vi "Differential IO.vi"(8 "error in (no error)":errorcluster, 11 "Node Ptr":T4 format="%.0x") -> (0 "error out":errorcluster)   [LabVIEW 2016, in "DCM System Explorer.lvlib"]
uses:
  DCM System Explorer.lvlib
  <vilib>/NI Veristand/Custom Device API/Custom Device Item Ref.ctl
  <vilib>/Powertrain Controls/Device Drivers/DCM/Diff IO/RT/Setup.ctl
  <vilib>/Powertrain Controls/Device Drivers/DCM/Diff IO/FPGA/Mode.ctl
  <vilib>/Powertrain Controls/Device Drivers/DCM/Diff IO/RT/Angle Control.ctl
  Shared/DCM Properties.vi
  <vilib>/NI Veristand/Custom Device API/Get Item Property (String Array).vi
  <vilib>/NI Veristand/Custom Device API/Get Item Property (Double Array).vi
  Shared/DCM Constants and GUIDs.vi
  <vilib>/NI Veristand/Custom Device API/Set Item Property (String Array).vi
  <vilib>/NI Veristand/Custom Device API/Set Item Property (Double Array).vi
  <vilib>/NI VeriStand/Custom Device API/Custom Device API.lvlib
  DCM Shared.lvlib
  <vilib>/Powertrain Controls/Device Drivers/DCM/Diff IO/FPGA/DCM - FPGA - Diff IO.lvlib
  <vilib>/Powertrain Controls/Device Drivers/DCM/Diff IO/RT/DCM - RT - Diff IO.lvlib
panel:
  in  "Digital filter [s]":sgl format="%#_2p"
  in  "Filters":sgl[](array[numeric])
  in  "_Setup Element":T1={"Mode"=enum."Off", "Capture Start [DBTDC]"=0.0, "Capture End [DBTDC]"=0.0, "Invert"=FALSE, "Frequency [Hz]"=0.0, "Duty Cycle [%]"=0.0, "TDC Offset [CAD]"=0.0, "Window Start [DBTDC]"=0.0, "Window End [DBTDC]"=0.0, "Angles"=[{"Enable"=FALSE, "Location [DBTDC]"=0.0, "Duration [s]"=0.0}, {"Enable"=FALSE, "Location [DBTDC]"=0.0, "Duration [s]"=0.0}, {"Enable"=FALSE, "Location [DBTDC]"=0.0, "Duration [s]"=0.0}, {"Enable"=FALSE, "Location [DBTDC]"=0.0, "Duration [s]"=0.0}], "Skip Fire"=FALSE, "Skip Fire Index"=0} caption="Command Setup" {"Skip Fire Index" max=7; "Angles"."Duration [s]" format="%#_3p"; "Frequency [Hz]" format="%#_3p"}
  in  "_Refresh":bool
  in  "Channel Names":string[](array[string])=["", "", "", "", "", "", "", "", "", "", "", ""]
  in  "Channel Name":string
  in  "_DiffIO Channels":i32[](listbox) caption="Channel Summary"
  in  "_Save Changes?":bool
  in  "Setup":T1[](array[typedef]) caption="Differential I/O Setup" {"Skip Fire Index" max=7; "Angles"."Duration [s]" format="%#_3p"; "Frequency [Hz]" format="%#_3p"}
  in  "Header":cluster{"Section Name":string}={"Section Name"="Differential I/O Initial Settings"}
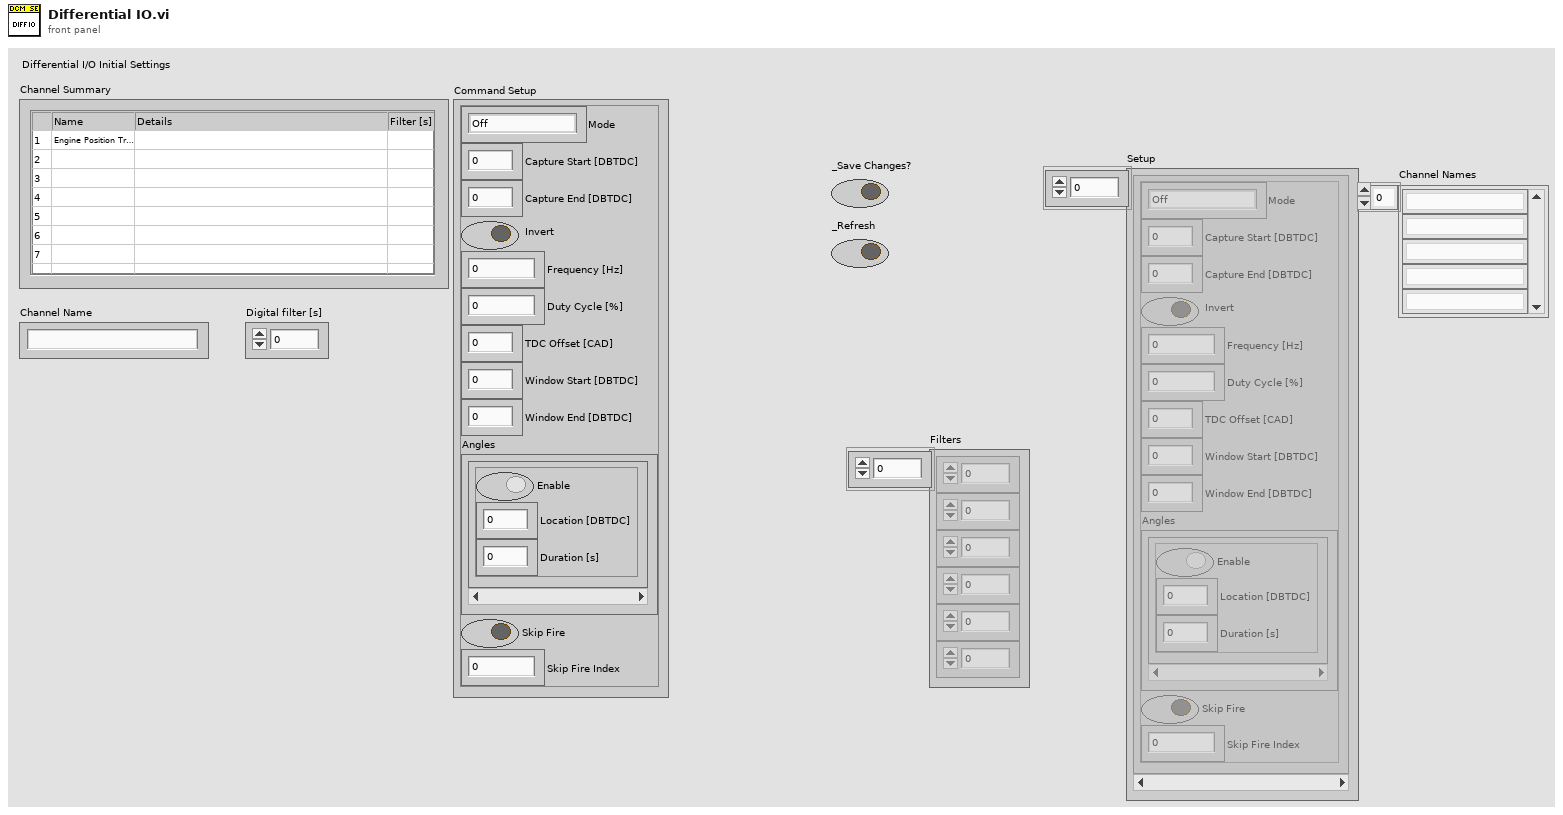
[diagram p1: front panel]
types:
  T1 = typedef "DCM - RT - Diff IO.lvlib/Setup.ctl" = cluster{"Mode":T2, "Capture Start [DBTDC]":sgl, "Capture End [DBTDC]":sgl, "Invert":bool, "Frequency [Hz]":sgl, "Duty Cycle [%]":sgl, "TDC Offset [CAD]":sgl, "Window Start [DBTDC]":sgl, "Window End [DBTDC]":sgl, "Angles":T3[], "Skip Fire":bool, "Skip Fire Index":u8}
  T2 = typedef "DCM - FPGA - Diff IO.lvlib/Mode.ctl" = enum8{"Off", "Input", "Pulse Width Modulation", "Engine Position Tracking", "Serial Out 1", "Serial Out 2", "EPTx Sync"}
  T3 = typedef "DCM - RT - Diff IO.lvlib/Angle Control.ctl" = cluster{"Enable":bool, "Location [DBTDC]":sgl, "Duration [s]":sgl}
  T4 = typedef "Custom Device API.lvlib/Custom Device Item Ref.ctl" = u64
  T5 = typedef "Custom Device API.lvlib/Custom Device Commands.ctl" = enum16{"Default", "Item renamed", "Shutdown", "Dynamic button pressed"}
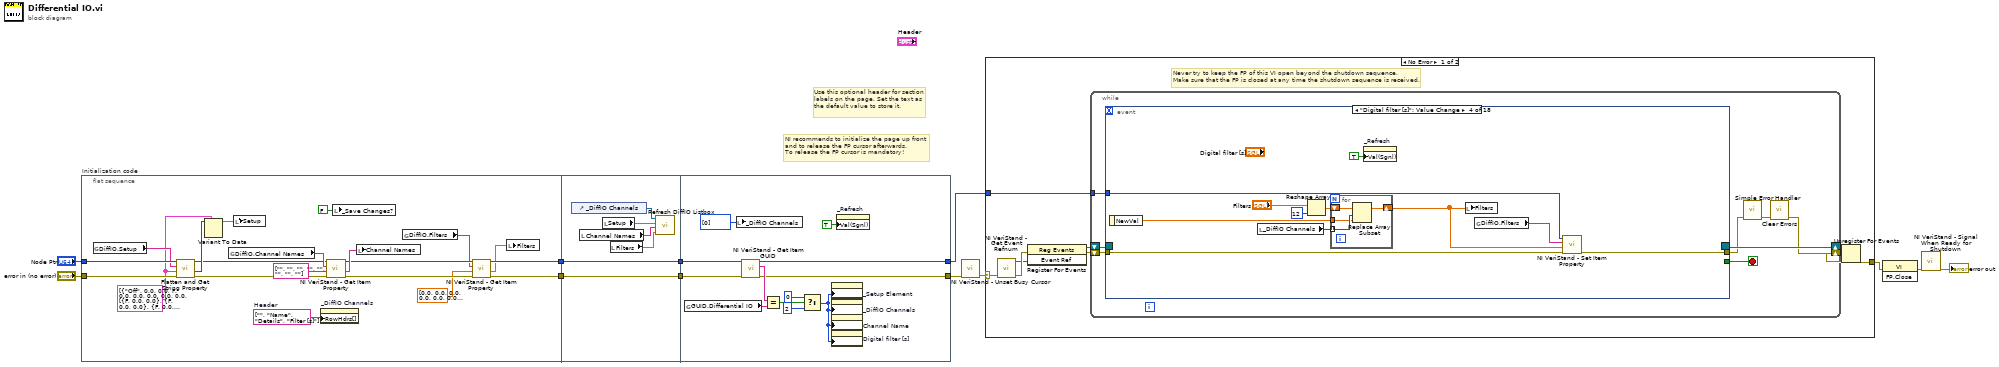
[diagram p0: block diagram]
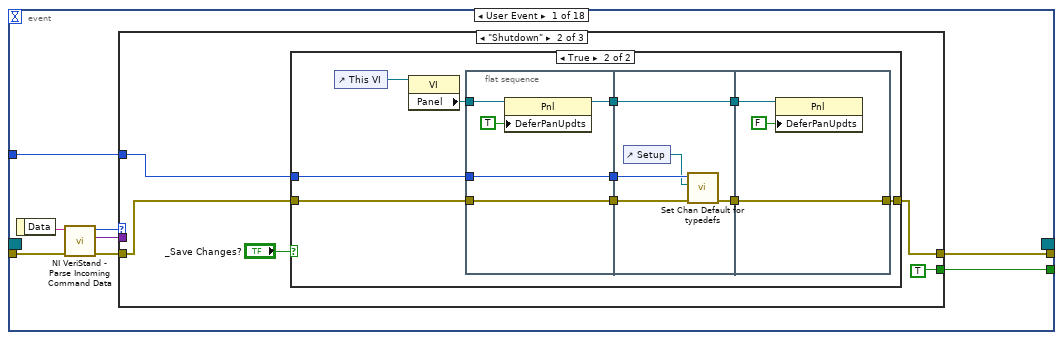
[diagram p2: hidden frame]
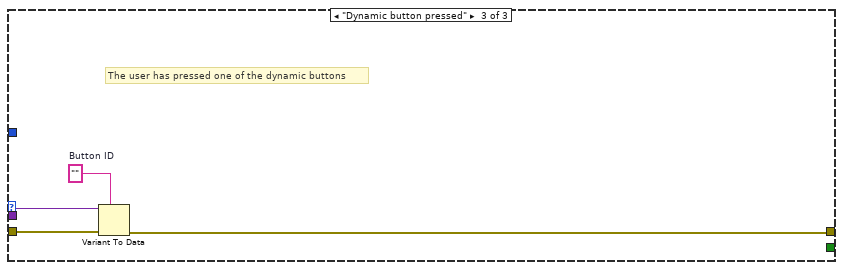
[diagram p5: hidden frame]
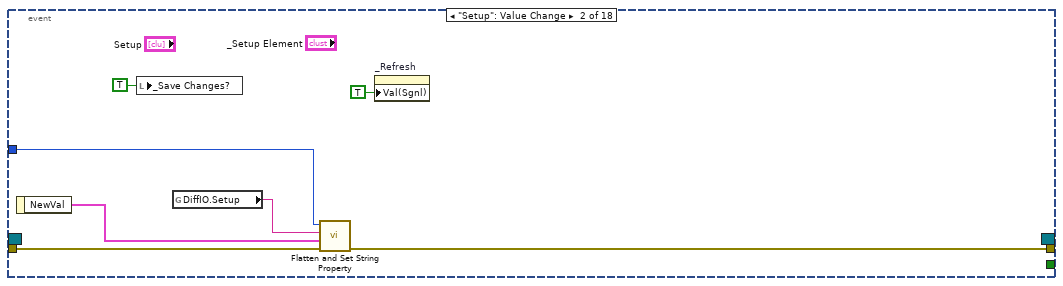
[diagram p6: hidden frame]
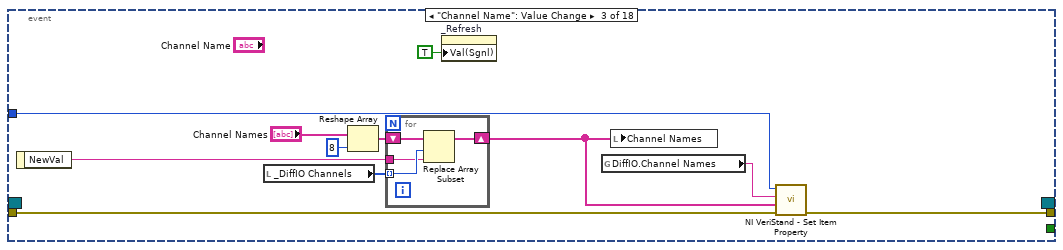
[diagram p7: hidden frame]
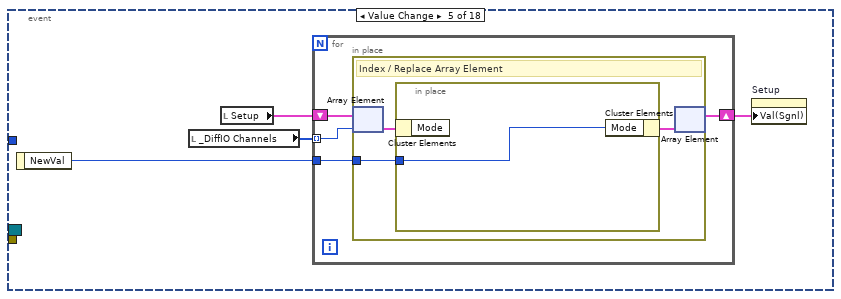
[diagram p8: hidden frame]
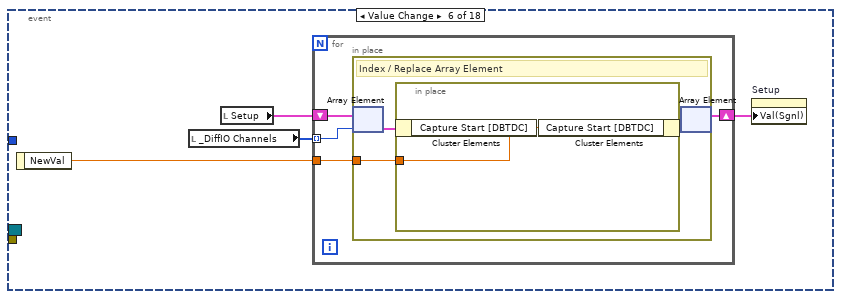
[diagram p9: hidden frame]
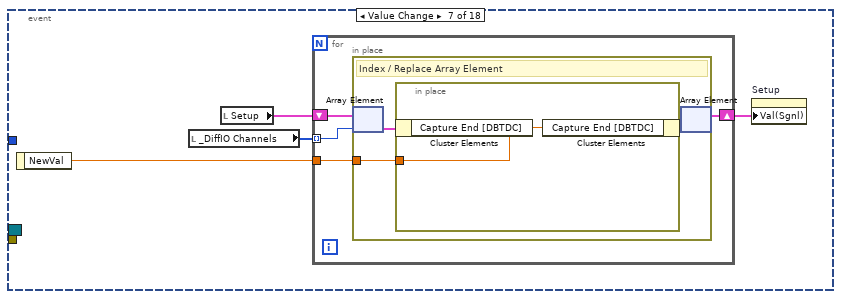
[diagram p10: hidden frame]
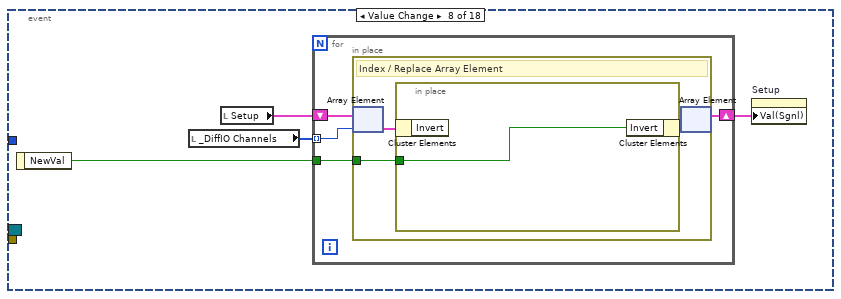
[diagram p11: hidden frame]
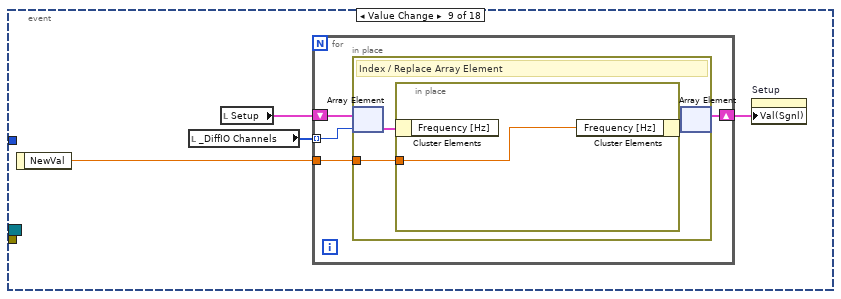
[diagram p12: hidden frame]
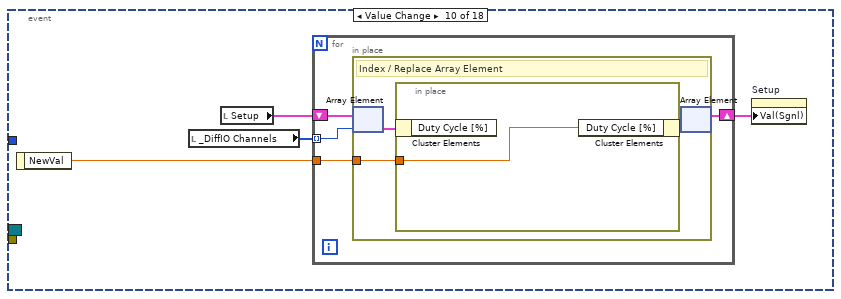
[diagram p13: hidden frame]
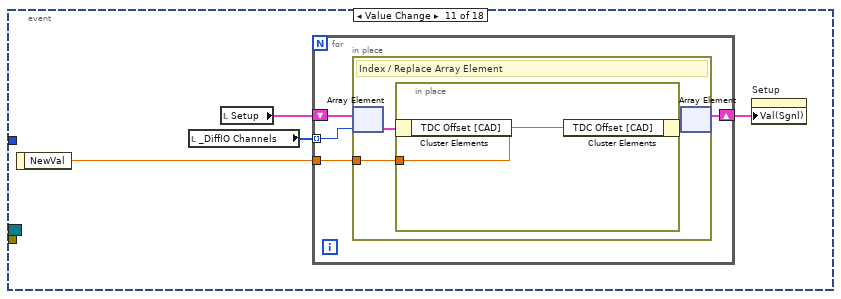
[diagram p14: hidden frame]
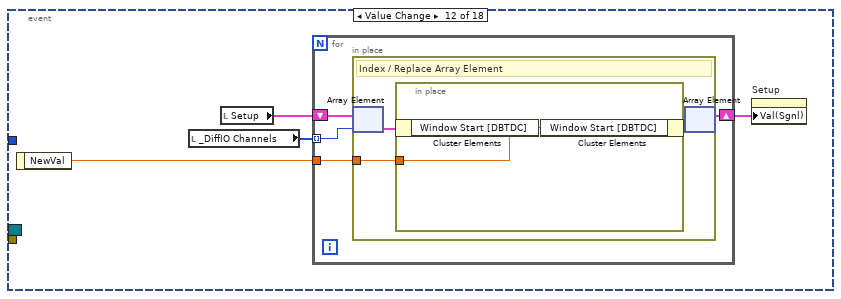
[diagram p15: hidden frame]
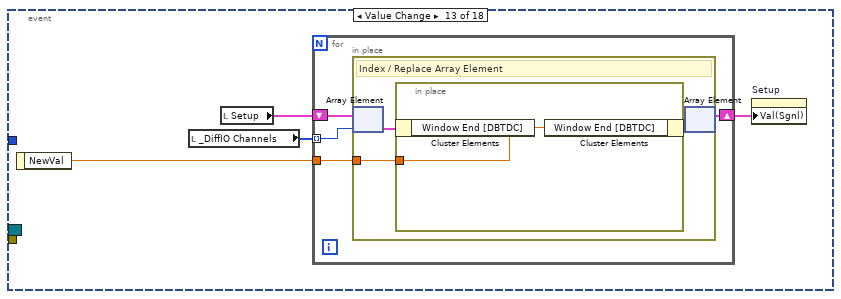
[diagram p16: hidden frame]
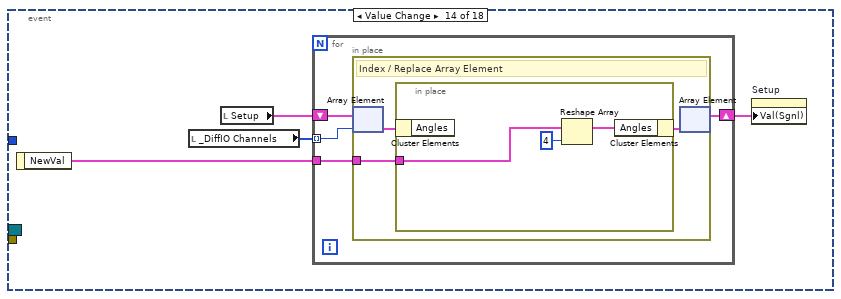
[diagram p17: hidden frame]
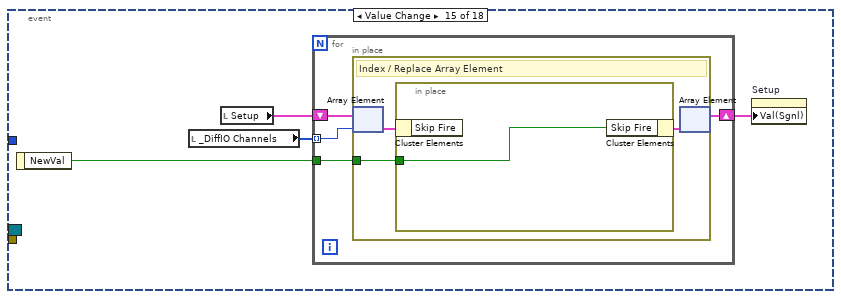
[diagram p18: hidden frame]
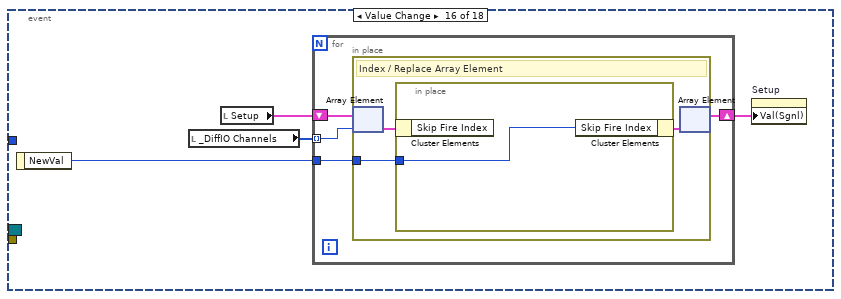
[diagram p19: hidden frame]
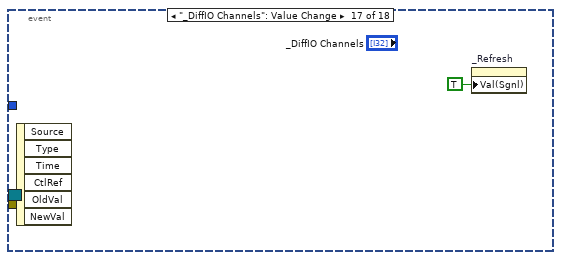
[diagram p20: hidden frame]
diagram:
  # "Use this optional header for section labels on the page. Set the text as the default value to store it."
  # "NI recommends to initialize the page up front\nand to release the FP cursor afterwards.\nTo release the FP cursor is mandatory!"
  n1 = flat-sequence "Initialization code" {
    tunnel: "Node Ptr" -> [w30]
    tunnel: "error in (no error)" -> [w31]
    tunnel: [w17] -> w5
    tunnel: [w16] -> w1
    tunnel: w5 -> [w37]
    tunnel: [w38] -> w4
    tunnel: [w37] -> w3
    tunnel: w1 -> [w38]
    tunnel: [w43] -> w2
    tunnel: [w42] -> w6
    tunnel: w4 -> [w45]
    tunnel: w3 -> [w44]
    frame #0 {
      w22 = string[] ["", "Name", "Details", "Filter [s]"]  # Header
      w28 = T1[] [{"Mode"=enum."Off", "Capture Start [DBTDC]"=0.0, "Capture End [DBTDC]"=0.0, "Invert"=FALSE, "Frequency [Hz]"=0.0, "Duty Cycle [%]"=0.0, "TDC Offset [CAD]"=0.0, "Window Start [DBTDC]"=0.0, "Window End [DBTDC]"=0.0, "Angles"=[{"Enable"=FALSE, "Location [DBTDC]"=0.0, "Duration [s]"=0.0}, {"Enable"=FALSE, "Location [DBTDC]"=0.0, "Duration [s]"=0.0}, {"Enable"=FALSE, "Location [DBTDC]"=0.0, "Duration [s]"=0.0}, {"Enable"=FALSE, "Location [DBTDC]"=0.0, "Duration [s]"=0.0}], "Skip Fire"=FALSE, "Skip Fire Index"=0}, {"Mode"=enum."Off", "Capture Start [DBTDC]"=0.0, "Capture End [DBTDC]"=0.0, "Invert"=FALSE, "Frequency [Hz]"=0.0, "Duty Cycle [%]"=0.0, "TDC Offset [CAD]"=0.0, "Window Start [DBTDC]"=0.0, "Window End [DBTDC]"=0.0, "Angles"=[{"Enable"=FALSE, "Location [DBTDC]"=0.0, "Duration [s]"=0.0}, {"Enable"=FALSE, "Location [DBTDC]"=0.0, "Duration [s]"=0.0}, {"Enable"=FALSE, "Location [DBTDC]"=0.0, "Duration [s]"=0.0}, {"Enable"=FALSE, "Location [DBTDC]"=0.0, "Duration [s]"=0.0}], "Skip Fire"=FALSE, "Skip Fire Index"=0}, {"Mode"=enum."Off", "Capture Start [DBTDC]"=0.0, "Capture End [DBTDC]"=0.0, "Invert"=FALSE, "Frequency [Hz]"=0.0, "Duty Cycle [%]"=0.0, "TDC Offset [CAD]"=0.0, "Window Start [DBTDC]"=0.0, "Window End [DBTDC]"=0.0, "Angles"=[{"Enable"=FALSE, "Location [DBTDC]"=0.0, "Duration [s]"=0.0}, {"Enable"=FALSE, "Location [DBTDC]"=0.0, "Duration [s]"=0.0}, {"Enable"=FALSE, "Location [DBTDC]"=0.0, "Duration [s]"=0.0}, {"Enable"=FALSE, "Location [DBTDC]"=0.0, "Duration [s]"=0.0}], "Skip Fire"=FALSE, "Skip Fire Index"=0}, {"Mode"=enum."Off", "Capture Start [DBTDC]"=0.0, "Capture End [DBTDC]"=0.0, "Invert"=FALSE, "Frequency [Hz]"=0.0, "Duty Cycle [%]"=0.0, "TDC Offset [CAD]"=0.0, "Window Start [DBTDC]"=0.0, "Window End [DBTDC]"=0.0, "Angles"=[{"Enable"=FALSE, "Location [DBTDC]"=0.0, "Duration [s]"=0.0}, {"Enable"=FALSE, "Location [DBTDC]"=0.0, "Duration [s]"=0.0}, {"Enable"=FALSE, "Location [DBTDC]"=0.0, "Duration [s]"=0.0}, {"Enable"=FALSE, "Location [DBTDC]"=0.0, "Duration [s]"=0.0}], "Skip Fire"=FALSE, "Skip Fire Index"=0}, {"Mode"=enum."Off", "Capture Start [DBTDC]"=0.0, "Capture End [DBTDC]"=0.0, "Invert"=FALSE, "Frequency [Hz]"=0.0, "Duty Cycle [%]"=0.0, "TDC Offset [CAD]"=0.0, "Window Start [DBTDC]"=0.0, "Window End [DBTDC]"=0.0, "Angles"=[{"Enable"=FALSE, "Location [DBTDC]"=0.0, "Duration [s]"=0.0}, {"Enable"=FALSE, "Location [DBTDC]"=0.0, "Duration [s]"=0.0}, {"Enable"=FALSE, "Location [DBTDC]"=0.0, "Duration [s]"=0.0}, {"Enable"=FALSE, "Location [DBTDC]"=0.0, "Duration [s]"=0.0}], "Skip Fire"=FALSE, "Skip Fire Index"=0}, {"Mode"=enum."Off", "Capture Start [DBTDC]"=0.0, "Capture End [DBTDC]"=0.0, "Invert"=FALSE, "Frequency [Hz]"=0.0, "Duty Cycle [%]"=0.0, "TDC Offset [CAD]"=0.0, "Window Start [DBTDC]"=0.0, "Window End [DBTDC]"=0.0, "Angles"=[{"Enable"=FALSE, "Location [DBTDC]"=0.0, "Duration [s]"=0.0}, {"Enable"=FALSE, "Location [DBTDC]"=0.0, "Duration [s]"=0.0}, {"Enable"=FALSE, "Location [DBTDC]"=0.0, "Duration [s]"=0.0}, {"Enable"=FALSE, "Location [DBTDC]"=0.0, "Duration [s]"=0.0}], "Skip Fire"=FALSE, "Skip Fire Index"=0}, {"Mode"=enum."Off", "Capture Start [DBTDC]"=0.0, "Capture End [DBTDC]"=0.0, "Invert"=FALSE, "Frequency [Hz]"=0.0, "Duty Cycle [%]"=0.0, "TDC Offset [CAD]"=0.0, "Window Start [DBTDC]"=0.0, "Window End [DBTDC]"=0.0, "Angles"=[{"Enable"=FALSE, "Location [DBTDC]"=0.0, "Duration [s]"=0.0}, {"Enable"=FALSE, "Location [DBTDC]"=0.0, "Duration [s]"=0.0}, {"Enable"=FALSE, "Location [DBTDC]"=0.0, "Duration [s]"=0.0}, {"Enable"=FALSE, "Location [DBTDC]"=0.0, "Duration [s]"=0.0}], "Skip Fire"=FALSE, "Skip Fire Index"=0}, {"Mode"=enum."Off", "Capture Start [DBTDC]"=0.0, "Capture End [DBTDC]"=0.0, "Invert"=FALSE, "Frequency [Hz]"=0.0, "Duty Cycle [%]"=0.0, "TDC Offset [CAD]"=0.0, "Window Start [DBTDC]"=0.0, "Window End [DBTDC]"=0.0, "Angles"=[{"Enable"=FALSE, "Location [DBTDC]"=0.0, "Duration [s]"=0.0}, {"Enable"=FALSE, "Location [DBTDC]"=0.0, "Duration [s]"=0.0}, {"Enable"=FALSE, "Location [DBTDC]"=0.0, "Duration [s]"=0.0}, {"Enable"=FALSE, "Location [DBTDC]"=0.0, "Duration [s]"=0.0}], "Skip Fire"=FALSE, "Skip Fire Index"=0}] ("DiffIO.Setup")
      n2 = global read "DCM Properties.vi" "DiffIO.Setup"() -> (w29:string)
      n3 = call "Flatten and Get String Property.vi"("error in (no error)"=w31, "Default Value"=w28, "Property Name"=w29, "Section Ref in"=w30) -> ("error out"=w20:errorcluster, "Value"=w32:variant, "Section Ref out"=w21:T4)  [unwired: 5 in]
      n4 = Variant To Data(type=w28, Variant=w32) -> (data=w27:T1[])  [unwired: 1 in, 1 out]
      n5 = global read "DCM Properties.vi" "DiffIO.Channel Names"() -> (w25:string)
      n6 = local write "Setup"(w27) -> ()
      n7 = property on="_DiffIO Channels" class="MCListbox (strict)"("RowHdrs[]"=w22) -> ()  [unwired: 2 in, 2 out]
      n8 = call-poly <vilib>:"NI VeriStand - Get Item Property.vi"("error in (no error)"=w20, "Default Value"=string[] ["", "", "", "", "", "", "", ""], "Property Name"=w25, "Item Ref in"=w21) -> ("error out"=w18:errorcluster, "Value"=w24:string[], "Item Ref out"=w19:T4)  [unwired: 4 in, 1 out]
      n9 = local write "_Save Changes?"(FALSE ("_Save Changes?")) -> ()
      n10 = local write "Channel Names"(w24) -> ()
      n11 = global read "DCM Properties.vi" "DiffIO.Filters"() -> (w15:string)
      n12 = call-poly <vilib>:"NI VeriStand - Get Item Property.vi"("error in (no error)"=w18, "Default Value"=sgl[] [0.0, 0.0, 0.0, 0.0, 0.0, 0.0, 0.0, 0.0] ("Settings.Diff IO Filters [s]"), "Property Name"=w15, "Item Ref in"=w19) -> ("error out"=w17:errorcluster, "Value"=w13:dbl[], "Item Ref out"=w16:T4)  [unwired: 4 in, 1 out]
      n13 = local write "Filters"(w13) -> ()
    }
    frame #1 {
      n14 = control-ref of="_DiffIO Channels"() -> (w36:refnum<vi>)
      n15 = local read "Channel Names"() -> (w34:string[])
      n16 = local read "Setup"() -> (w35:T1[])
      n17 = local read "Filters"() -> (w33:sgl[])
      n18 = call "Refresh DiffIO Listbox.vi"("Filters"=w33, "Names"=w34, "Setup"=w35, "MulticolumnListbox in"=w36) -> ()  [unwired: 8 in]
    }
    frame #2 {
      n19 = global read "DCM Constants and GUIDs.vi" "GUID.Differential IO"() -> (w49:string)
      n20 = local write "_DiffIO Channels"(i32[] [0] ("_DiffIO Channels")) -> ()
      n21 = call <vilib>:"NI VeriStand - Get Item GUID.vi"("error in (no error)"=w44, "Item Ref in"=w45) -> ("error out"=w43:errorcluster, "GUID"=w48:string, "Item Ref out"=w42:T4)  [unwired: 7 in]
      n22 = Equal?(x=w48, y=w49) -> (x = y?=w50:bool)
      n23 = Select(t=0, s=w50, f=2) -> (s? t:f=w41:i32)
      n24 = property on="_Setup Element" class="Clust (strict)"("DisabledEnum"=w41) -> ()  [unwired: 2 in, 2 out]
      n25 = property on="_DiffIO Channels" class="MCListbox (strict)"("DisabledEnum"=w41) -> ()  [unwired: 2 in, 2 out]
      n26 = property on="Channel Name" class="Str"("DisabledEnum"=w41) -> ()  [unwired: 2 in, 2 out]
      n27 = property on="Digital filter [s]" class="DigNum (strict)"("DisabledEnum"=w41) -> ()  [unwired: 2 in, 2 out]
      n28 = property on="_Refresh" class="Bool (strict)"("Val(Sgnl)"=TRUE ("Value (Signaling)")) -> ()  [unwired: 2 in, 2 out]
    }
  }
  n29 = call <vilib>:"NI VeriStand - Unset Busy Cursor.vi"("error in (no error)"=w2) -> ("error out"=w8:errorcluster)  [unwired: 10 out]
  n30 = case shown="No Error" w8 {
    selector: w8 -> [w52 w310]
    tunnel: [w56 w308] -> w12
    tunnel: w6 -> [w51 _]
    frame No Error {
      # "Never try to keep the FP of this VI open beyond the shutdown sequence.\nMake sure that the FP is closed at any time the shutdown sequence is received."
      n31 = call <vilib>:"NI VeriStand - Get Event Refnum.vi"("error in (no error)"=w52) -> ("error out"=w59:errorcluster, "Event Ref"=w55:refnum<user-event>)  [unwired: 9 out]
      n32 = register-events(error in=w59, w55) -> (reference out=w53:refnum<event-registration>, error out=w54:errorcluster)  [unwired: 1 in]
      n33 = while {
        shift-right: [w61] -> w57
        shift-left: w54 -> [w66]
        shift-right: [w67] -> w58
        shift-left: w53 -> [w65]
        tunnel: w51 -> [w60]
        stop <- w64 stop-if-true
        n34 = event shown="[3] \"Digital filter [s]\": Value Change" {
          selector: w65 -> [_ _ _ _ _ _ _ _ _ _ _ _ _ _ _ _ _ _]
          dyn-events: [_ _ _ _ _ _ _ _ _ _ _ _ _ _ _ _ _ _] -> w67
          timeout: _ -> [_ _ _ _ _ _ _ _ _ _ _ _ _ _ _ _ _ _]
          tunnel: w66 -> [w75 w116 w127 w142 _ _ _ _ _ _ _ _ _ _ _ _ _ _]
          tunnel: [w71 _ _ _ _ _ _ _ _ _ _ _ _ _ _ _ _ _] -> w64
          tunnel: [w70 w115 w126 w141 _ _ _ _ _ _ _ _ _ _ _ _ _ _] -> w63
          tunnel: w60 -> [w68 w112 w124 w139 _ _ _ _ _ _ _ _ _ _ _ _ _ _]
          event User Event {
            n35 = event-data() -> ("Data"=w74:string)  [unwired: 1 out]
            n36 = call <vilib>:"NI VeriStand - Parse Incoming Command Data.vi"("error in (no error)"=w75, "Incoming data"=w74) -> ("error out"=w73:errorcluster, "Outgoing data"=w69:variant, "Action"=w72:T5)  [unwired: 7 out]
            n37 = case shown="\"Shutdown\"" w72 {
              tunnel: w73 -> [w76 w79 w109]
              tunnel: [_ TRUE _] -> w71
              tunnel: [w76 w78 w106] -> w70
              tunnel: w69 -> [_ _ w108]
              tunnel: w68 -> [_ w80 _]
              frame "Default", Default {
              }
              frame "Shutdown" {
                n38 = case shown="True" "_Save Changes?" {
                  tunnel: w80 -> [_ w87]
                  tunnel: w79 -> [w82 w86]
                  tunnel: [w82 w85] -> w78
                  frame False {
                  }
                  frame True {
                    n39 = control-ref of="This VI"() -> (w84:refnum<vi>)
                    n40 = property class="VI"(reference=w84) -> ("Panel"=w83:refnum<vi>)  [unwired: 1 in, 2 out]
                    n41 = flat-sequence {
                      tunnel: w86 -> [w96]
                      tunnel: w87 -> [w97]
                      tunnel: [w97] -> w92
                      tunnel: [w96] -> w91
                      tunnel: w83 -> [w95]
                      tunnel: [w93] -> w90
                      tunnel: w92 -> [w102]
                      tunnel: w91 -> [w101]
                      tunnel: [w100] -> w89
                      tunnel: [w99] -> w88
                      tunnel: w90 -> [w99]
                      tunnel: [w105] -> w85
                      tunnel: w89 -> [w105]
                      tunnel: w88 -> [w103]
                      frame #0 {
                        n42 = property class="Pnl"(reference=w95, "DeferPanUpdts"=TRUE ("Defer Panel Updates")) -> (reference out=w93:refnum<vi>)  [unwired: 1 in, 1 out]
                      }
                      frame #1 {
                        n43 = control-ref of="Setup"() -> (w98:refnum<vi>)
                        n44 = call "Set Chan Default for typedefs.vi"("error in"=w101, "Ctl Ref"=w98, "Section Ref in"=w102) -> ("error out"=w100:errorcluster)  [unwired: 7 in, 1 out]
                      }
                      frame #2 {
                        n45 = property class="Pnl"(reference=w103, "DeferPanUpdts"=FALSE ("Defer Panel Updates")) -> ()  [unwired: 1 in, 2 out]
                      }
                    }
                  }
                }
              }
              frame "Dynamic button pressed" {
                w107 = ""  # Button ID
                # "The user has pressed one of the dynamic buttons"
                n46 = Variant To Data(error in=w109, type=w107, Variant=w108) -> (error out=w106:errorcluster)  [unwired: 1 out]
              }
            }
          }
          event "Setup": Value Change {
            n47 = event-data() -> ("NewVal"=w113:T1[])  [unwired: 1 out]
            n48 = local write "_Save Changes?"(TRUE ("_Save Changes?")) -> ()
            n49 = global read "DCM Properties.vi" "DiffIO.Setup"() -> (w114:string)
            n50 = call "Flatten and Set String Property.vi"("error in (no error)"=w116, "Value"=w113, "Property Name"=w114, "Section Ref in"=w112) -> ("error out"=w115:errorcluster)  [unwired: 6 in, 1 out]
            n51 = property on="_Refresh" class="Bool (strict)"("Val(Sgnl)"=TRUE ("Value (Signaling)")) -> ()  [unwired: 2 in, 2 out]
          }
          event "Channel Name": Value Change {
            n52 = event-data() -> ("NewVal"=w120:string)  [unwired: 1 out]
            n53 = local read "_DiffIO Channels"() -> (w121:i32[])
            n54 = Reshape Array("Channel Names", 8 ("dimension size")) -> (w123:string[])
            n55 = for {
              tunnel: w121 -> [w129] mode=indexing
              shift-right: [w130] -> w117
              shift-left: w123 -> [w131]
              tunnel: w120 -> [w128]
              n56 = Replace Array Subset(array=w131, new element=w128, index=w129) -> (w130:string[])
            }
            n57 = property on="_Refresh" class="Bool (strict)"("Val(Sgnl)"=TRUE ("Value (Signaling)")) -> ()  [unwired: 2 in, 2 out]
            n58 = global read "DCM Properties.vi" "DiffIO.Channel Names"() -> (w125:string)
            n59 = local write "Channel Names"(w117) -> ()
            n60 = call-poly <vilib>:"NI VeriStand - Set Item Property.vi"("error in (no error)"=w127, "Value"=w117, "Property Name"=w125, "Item Ref in"=w124) -> ("error out"=w126:errorcluster)  [unwired: 5 in, 2 out]
          }
          event "Digital filter [s]": Value Change {
            n61 = event-data() -> ("NewVal"=w135:sgl)  [unwired: 1 out]
            n62 = local read "_DiffIO Channels"() -> (w136:i32[])
            n63 = Reshape Array("Filters", 12 ("dimension size")) -> (w138:sgl[])
            n64 = for {
              tunnel: w136 -> [w144] mode=indexing
              shift-right: [w145] -> w132
              shift-left: w138 -> [w146]
              tunnel: w135 -> [w143]
              n65 = Replace Array Subset(array=w146, new element=w143, index=w144) -> (w145:sgl[])
            }
            n66 = property on="_Refresh" class="Bool (strict)"("Val(Sgnl)"=TRUE ("Value (Signaling)")) -> ()  [unwired: 2 in, 2 out]
            n67 = local write "Filters"(w132) -> ()
            n68 = global read "DCM Properties.vi" "DiffIO.Filters"() -> (w140:string)
            n69 = call-poly <vilib>:"NI VeriStand - Set Item Property.vi"("error in (no error)"=w142, "Value"=w132, "Property Name"=w140, "Item Ref in"=w139) -> ("error out"=w141:errorcluster)  [unwired: 5 in, 2 out]
          }
          event Value Change {
            n70 = event-data() -> ("NewVal"=w147:T2)  [unwired: 1 out]
            n71 = local read "_DiffIO Channels"() -> (w148:i32[])
            n72 = local read "Setup"() -> (w149:T1[])
            n73 = for {
              tunnel: w148 -> [w153] mode=indexing
              shift-right: [w152] -> w150
              shift-left: w149 -> [w154]
              tunnel: w147 -> [w151]
              n74 = in-place {
                in-place-border: w151 -> [w155]
                # "Index / Replace Array Element"
                n75 = in-place-array #1(w154, w153) -> (w157:T1)
                n76 = in-place {
                  in-place-border: w155 -> [w158]
                  n77 = in-place-cluster #2(w157) -> ()  [unwired: 1 out]
                  n78 = in-place-cluster #2("Mode"=w158) -> (w156:T1)
                }
                n79 = in-place-array #1(w156) -> (w152:T1[])  [unwired: 1 out]
              }
            }
            n80 = property on="Setup" class="Arr (strict)"("Val(Sgnl)"=w150) -> ()  [unwired: 2 in, 2 out]
          }
          event Value Change {
            n81 = event-data() -> ("NewVal"=w159:sgl)  [unwired: 1 out]
            n82 = local read "_DiffIO Channels"() -> (w160:i32[])
            n83 = local read "Setup"() -> (w161:T1[])
            n84 = for {
              tunnel: w160 -> [w165] mode=indexing
              shift-right: [w164] -> w162
              shift-left: w161 -> [w166]
              tunnel: w159 -> [w163]
              n85 = in-place {
                in-place-border: w163 -> [w167]
                # "Index / Replace Array Element"
                n86 = in-place-array #3(w166, w165) -> (w169:T1)
                n87 = in-place {
                  in-place-border: w167 -> [w170]
                  n88 = in-place-cluster #4(w169) -> ()  [unwired: 1 out]
                  n89 = in-place-cluster #4("Capture Start [DBTDC]"=w170) -> (w168:T1)
                }
                n90 = in-place-array #3(w168) -> (w164:T1[])  [unwired: 1 out]
              }
            }
            n91 = property on="Setup" class="Arr (strict)"("Val(Sgnl)"=w162) -> ()  [unwired: 2 in, 2 out]
          }
          event Value Change {
            n92 = event-data() -> ("NewVal"=w171:sgl)  [unwired: 1 out]
            n93 = local read "_DiffIO Channels"() -> (w172:i32[])
            n94 = local read "Setup"() -> (w173:T1[])
            n95 = for {
              tunnel: w172 -> [w177] mode=indexing
              shift-right: [w176] -> w174
              shift-left: w173 -> [w178]
              tunnel: w171 -> [w175]
              n96 = in-place {
                in-place-border: w175 -> [w179]
                # "Index / Replace Array Element"
                n97 = in-place-array #5(w178, w177) -> (w181:T1)
                n98 = in-place {
                  in-place-border: w179 -> [w182]
                  n99 = in-place-cluster #6(w181) -> ()  [unwired: 1 out]
                  n100 = in-place-cluster #6("Capture End [DBTDC]"=w182) -> (w180:T1)
                }
                n101 = in-place-array #5(w180) -> (w176:T1[])  [unwired: 1 out]
              }
            }
            n102 = property on="Setup" class="Arr (strict)"("Val(Sgnl)"=w174) -> ()  [unwired: 2 in, 2 out]
          }
          event Value Change {
            n103 = event-data() -> ("NewVal"=w183:bool)  [unwired: 1 out]
            n104 = local read "_DiffIO Channels"() -> (w184:i32[])
            n105 = local read "Setup"() -> (w185:T1[])
            n106 = for {
              tunnel: w184 -> [w189] mode=indexing
              shift-right: [w188] -> w186
              shift-left: w185 -> [w190]
              tunnel: w183 -> [w187]
              n107 = in-place {
                in-place-border: w187 -> [w191]
                # "Index / Replace Array Element"
                n108 = in-place-array #7(w190, w189) -> (w193:T1)
                n109 = in-place {
                  in-place-border: w191 -> [w194]
                  n110 = in-place-cluster #8(w193) -> ()  [unwired: 1 out]
                  n111 = in-place-cluster #8("Invert"=w194) -> (w192:T1)
                }
                n112 = in-place-array #7(w192) -> (w188:T1[])  [unwired: 1 out]
              }
            }
            n113 = property on="Setup" class="Arr (strict)"("Val(Sgnl)"=w186) -> ()  [unwired: 2 in, 2 out]
          }
          event Value Change {
            n114 = event-data() -> ("NewVal"=w195:sgl)  [unwired: 1 out]
            n115 = local read "_DiffIO Channels"() -> (w196:i32[])
            n116 = local read "Setup"() -> (w197:T1[])
            n117 = for {
              tunnel: w196 -> [w201] mode=indexing
              shift-right: [w200] -> w198
              shift-left: w197 -> [w202]
              tunnel: w195 -> [w199]
              n118 = in-place {
                in-place-border: w199 -> [w203]
                # "Index / Replace Array Element"
                n119 = in-place-array #9(w202, w201) -> (w205:T1)
                n120 = in-place {
                  in-place-border: w203 -> [w206]
                  n121 = in-place-cluster #10(w205) -> ()  [unwired: 1 out]
                  n122 = in-place-cluster #10("Frequency [Hz]"=w206) -> (w204:T1)
                }
                n123 = in-place-array #9(w204) -> (w200:T1[])  [unwired: 1 out]
              }
            }
            n124 = property on="Setup" class="Arr (strict)"("Val(Sgnl)"=w198) -> ()  [unwired: 2 in, 2 out]
          }
          event Value Change {
            n125 = event-data() -> ("NewVal"=w207:sgl)  [unwired: 1 out]
            n126 = local read "_DiffIO Channels"() -> (w208:i32[])
            n127 = local read "Setup"() -> (w209:T1[])
            n128 = for {
              tunnel: w208 -> [w213] mode=indexing
              shift-right: [w212] -> w210
              shift-left: w209 -> [w214]
              tunnel: w207 -> [w211]
              n129 = in-place {
                in-place-border: w211 -> [w215]
                # "Index / Replace Array Element"
                n130 = in-place-array #11(w214, w213) -> (w217:T1)
                n131 = in-place {
                  in-place-border: w215 -> [w218]
                  n132 = in-place-cluster #12(w217) -> ()  [unwired: 1 out]
                  n133 = in-place-cluster #12("Duty Cycle [%]"=w218) -> (w216:T1)
                }
                n134 = in-place-array #11(w216) -> (w212:T1[])  [unwired: 1 out]
              }
            }
            n135 = property on="Setup" class="Arr (strict)"("Val(Sgnl)"=w210) -> ()  [unwired: 2 in, 2 out]
          }
          event Value Change {
            n136 = event-data() -> ("NewVal"=w219:sgl)  [unwired: 1 out]
            n137 = local read "_DiffIO Channels"() -> (w220:i32[])
            n138 = local read "Setup"() -> (w221:T1[])
            n139 = for {
              tunnel: w220 -> [w225] mode=indexing
              shift-right: [w224] -> w222
              shift-left: w221 -> [w226]
              tunnel: w219 -> [w223]
              n140 = in-place {
                in-place-border: w223 -> [w227]
                # "Index / Replace Array Element"
                n141 = in-place-array #13(w226, w225) -> (w229:T1)
                n142 = in-place {
                  in-place-border: w227 -> [w230]
                  n143 = in-place-cluster #14(w229) -> ()  [unwired: 1 out]
                  n144 = in-place-cluster #14("TDC Offset [CAD]"=w230) -> (w228:T1)
                }
                n145 = in-place-array #13(w228) -> (w224:T1[])  [unwired: 1 out]
              }
            }
            n146 = property on="Setup" class="Arr (strict)"("Val(Sgnl)"=w222) -> ()  [unwired: 2 in, 2 out]
          }
          event Value Change {
            n147 = event-data() -> ("NewVal"=w231:sgl)  [unwired: 1 out]
            n148 = local read "_DiffIO Channels"() -> (w232:i32[])
            n149 = local read "Setup"() -> (w233:T1[])
            n150 = for {
              tunnel: w232 -> [w237] mode=indexing
              shift-right: [w236] -> w234
              shift-left: w233 -> [w238]
              tunnel: w231 -> [w235]
              n151 = in-place {
                in-place-border: w235 -> [w239]
                # "Index / Replace Array Element"
                n152 = in-place-array #15(w238, w237) -> (w241:T1)
                n153 = in-place {
                  in-place-border: w239 -> [w242]
                  n154 = in-place-cluster #16(w241) -> ()  [unwired: 1 out]
                  n155 = in-place-cluster #16("Window Start [DBTDC]"=w242) -> (w240:T1)
                }
                n156 = in-place-array #15(w240) -> (w236:T1[])  [unwired: 1 out]
              }
            }
            n157 = property on="Setup" class="Arr (strict)"("Val(Sgnl)"=w234) -> ()  [unwired: 2 in, 2 out]
          }
          event Value Change {
            n158 = event-data() -> ("NewVal"=w243:sgl)  [unwired: 1 out]
            n159 = local read "_DiffIO Channels"() -> (w244:i32[])
            n160 = local read "Setup"() -> (w245:T1[])
            n161 = for {
              tunnel: w244 -> [w249] mode=indexing
              shift-right: [w248] -> w246
              shift-left: w245 -> [w250]
              tunnel: w243 -> [w247]
              n162 = in-place {
                in-place-border: w247 -> [w251]
                # "Index / Replace Array Element"
                n163 = in-place-array #17(w250, w249) -> (w253:T1)
                n164 = in-place {
                  in-place-border: w251 -> [w254]
                  n165 = in-place-cluster #18(w253) -> ()  [unwired: 1 out]
                  n166 = in-place-cluster #18("Window End [DBTDC]"=w254) -> (w252:T1)
                }
                n167 = in-place-array #17(w252) -> (w248:T1[])  [unwired: 1 out]
              }
            }
            n168 = property on="Setup" class="Arr (strict)"("Val(Sgnl)"=w246) -> ()  [unwired: 2 in, 2 out]
          }
          event Value Change {
            n169 = event-data() -> ("NewVal"=w255:T3[])  [unwired: 1 out]
            n170 = local read "_DiffIO Channels"() -> (w256:i32[])
            n171 = local read "Setup"() -> (w257:T1[])
            n172 = for {
              tunnel: w256 -> [w261] mode=indexing
              shift-right: [w260] -> w258
              shift-left: w257 -> [w262]
              tunnel: w255 -> [w259]
              n173 = in-place {
                in-place-border: w259 -> [w263]
                # "Index / Replace Array Element"
                n174 = in-place-array #19(w262, w261) -> (w265:T1)
                n175 = in-place {
                  in-place-border: w263 -> [w268]
                  n176 = in-place-cluster #20(w265) -> ()  [unwired: 1 out]
                  n177 = Reshape Array(w268, 4 ("dimension size")) -> (w267:T3[])
                  n178 = in-place-cluster #20("Angles"=w267) -> (w264:T1)
                }
                n179 = in-place-array #19(w264) -> (w260:T1[])  [unwired: 1 out]
              }
            }
            n180 = property on="Setup" class="Arr (strict)"("Val(Sgnl)"=w258) -> ()  [unwired: 2 in, 2 out]
          }
          event Value Change {
            n181 = event-data() -> ("NewVal"=w269:bool)  [unwired: 1 out]
            n182 = local read "_DiffIO Channels"() -> (w270:i32[])
            n183 = local read "Setup"() -> (w271:T1[])
            n184 = for {
              tunnel: w270 -> [w275] mode=indexing
              shift-right: [w274] -> w272
              shift-left: w271 -> [w276]
              tunnel: w269 -> [w273]
              n185 = in-place {
                in-place-border: w273 -> [w277]
                # "Index / Replace Array Element"
                n186 = in-place-array #21(w276, w275) -> (w279:T1)
                n187 = in-place {
                  in-place-border: w277 -> [w280]
                  n188 = in-place-cluster #22(w279) -> ()  [unwired: 1 out]
                  n189 = in-place-cluster #22("Skip Fire"=w280) -> (w278:T1)
                }
                n190 = in-place-array #21(w278) -> (w274:T1[])  [unwired: 1 out]
              }
            }
            n191 = property on="Setup" class="Arr (strict)"("Val(Sgnl)"=w272) -> ()  [unwired: 2 in, 2 out]
          }
          event Value Change {
            n192 = event-data() -> ("NewVal"=w281:u8)  [unwired: 1 out]
            n193 = local read "_DiffIO Channels"() -> (w282:i32[])
            n194 = local read "Setup"() -> (w283:T1[])
            n195 = for {
              tunnel: w282 -> [w287] mode=indexing
              shift-right: [w286] -> w284
              shift-left: w283 -> [w288]
              tunnel: w281 -> [w285]
              n196 = in-place {
                in-place-border: w285 -> [w289]
                # "Index / Replace Array Element"
                n197 = in-place-array #23(w288, w287) -> (w291:T1)
                n198 = in-place {
                  in-place-border: w289 -> [w292]
                  n199 = in-place-cluster #24(w291) -> ()  [unwired: 1 out]
                  n200 = in-place-cluster #24("Skip Fire Index"=w292) -> (w290:T1)
                }
                n201 = in-place-array #23(w290) -> (w286:T1[])  [unwired: 1 out]
              }
            }
            n202 = property on="Setup" class="Arr (strict)"("Val(Sgnl)"=w284) -> ()  [unwired: 2 in, 2 out]
          }
          event "_DiffIO Channels": Value Change {
            n203 = event-data() -> ()  [unwired: 7 out]
            n204 = property on="_Refresh" class="Bool (strict)"("Val(Sgnl)"=TRUE ("Value (Signaling)")) -> ()  [unwired: 2 in, 2 out]
          }
          event "_Refresh": Value Change {
            n205 = event-data() -> ()  [unwired: 7 out]
            n206 = local write "_Refresh"(FALSE ("_Refresh")) -> ()
            n207 = stacked-sequence {
              frame #0 {
                n208 = local read "_DiffIO Channels"() -> (w297:i32[])
                n209 = local read "Channel Names"() -> (w303:string[])
                n210 = local read "Setup"() -> (w301:T1[])
                n211 = local read "Filters"() -> (w299:sgl[])
                n212 = Index Array(array=w297, index=0) -> (element=w296:i32)
                n213 = Index Array(array=w301, index=w296) -> (element=w300:T1)
                n214 = Index Array(array=w303, index=w296) -> (element=w302:string)
                n215 = Index Array(array=w299, index=w296) -> (element=w298:sgl)
                n216 = local write "Channel Name"(w302) -> ()
                n217 = local write "Digital filter [s]"(w298) -> ()
                n218 = local write "_Setup Element"(w300) -> ()
              }
              frame #1 {
                n219 = control-ref of="_DiffIO Channels"() -> (w304:refnum<vi>)
                n220 = local read "Channel Names"() -> (w306:string[])
                n221 = local read "Filters"() -> (w305:sgl[])
                n222 = local read "Setup"() -> (w307:T1[])
                n223 = call "Refresh DiffIO Listbox.vi"("Filters"=w305, "Names"=w306, "Setup"=w307, "MulticolumnListbox in"=w304) -> ()  [unwired: 8 in]
              }
            }
          }
        }
        n224 = call <vilib>:"Simple Error Handler.vi"("error in (no error)"=w63) -> ("error out"=w62:errorcluster)  [unwired: 1 in, 7 out]
        n225 = call <vilib>:"Clear Errors.vi"("error in (no error)"=w62) -> ("error out"=w61:errorcluster)  [unwired: 1 in, 5 out]
      }
      n226 = Unregister For Events(event registration refnum=w58, error in=w57) -> (error out=w56:errorcluster)
    }
    frame Error {
      n227 = call <vilib>:"Simple Error Handler.vi"("error in (no error)"=w310) -> ("error out"=w309:errorcluster)  [unwired: 1 in, 7 out]
      n228 = call <vilib>:"Clear Errors.vi"("error in (no error)"=w309) -> ("error out"=w308:errorcluster)  [unwired: 1 in, 5 out]
    }
  }
  n229 = invoke class="VI" method="FP.Close"(error in=w12) -> (error out=w11:errorcluster)  [unwired: 2 in, 2 out]
  n230 = call <vilib>:"NI VeriStand - Signal When Ready for Shutdown.vi"("error in (no error)"=w11) -> ("error out"=→"error out":errorcluster)  [unwired: 10 out]
